vi "Current Loop - NI 9505 (FPGA).vi"() -> ()   [LabVIEW 2012]
doc: "This VI shows an example of how to implement a current loop for use with the NI 9505. The VI consists of a closed loop PI system with PWM generation and error monitoring. The desired load current can be set and the loop will monitor the actual current and adjust the PWM duty cycle until the desired current is reached."
uses:
  <vilib>/LabVIEW Targets/FPGA/cRIO/cRIO-9505/controls.llb/_nicrio_cRIO-9505_DriveStatus.ctl
  <vilib>/Platform/TimedLoop/XDataNode/timing_clust.ctl
  <vilib>/Platform/TimedLoop/XDataNode/nitl_modes.ctl
  <vilib>/Platform/TimedLoop/XDataNode/wakeup.ctl
  <vilib>/LabVIEW Targets/FPGA/cRIO/cRIO-9505/controls.llb/_nicrio_cRIO-9505_DriveDirection.ctl
  <vilib>/rvi/Emulation/niFpgaSctlEmulationRegisterWithScheduler.vi
  <vilib>/rvi/Emulation/niFpgaSctlEmulationScheduler.vi
  <vilib>/rvi/Emulation/niFpgaSctlEmulationGetInTimedLoop.vi
  <vilib>/rvi/eio/common/nirviEmuTemplateMethod_errors.vi
  <vilib>/rvi/Emulation/niFpgaSctlEmulationGlobalWrite.vi
  <vilib>/rvi/eio/common/nirviEmuTemplatePropertyGet_noerrors.vi
  Instance           1 37Saved   Current Loop - NI 9505 (FPGA) .vi
  <vilib>/Platform/TimedLoop/XDataNode/XDataNode.xnode
  <vilib>/eio/EIONode/EIONode.xnode
  <vilib>/eio/EIOMethodNode/EIOMethodNode.xnode
  <vilib>/eio/EIOPropertyNode/EIOPropertyNode.xnode
  <vilib>/Platform/TimedLoop/XDataNode/XDNodeRunTimeDep.lvlib
  <vilib>/rvi/eio/common/nirviEmuTemplatePropertyGet_errors.vi
  <vilib>/rvi/eio/common/nirviEmuTemplatePropertySet_errors.vi
  <vilib>/rvi/eio/common/nirviEmuTemplatePropertySet_noerrors.vi
panel:
  in  "Disable\nDrive":bool
  in  "Enable\nDrive":bool
  out "Temp Fault":bool
  out "Drive Status":T1=enum."Disabled"
  out "Drive Fault":bool
  out "Vsup Present":bool
  in  "Current Loop\nRate (usec)":u32=50
  in  "Current Limit":i16 caption="Setpoint" min=0 max=2047
  in  "Current PI gains":T2={"Proportional Gain"=20, "Integral Gain"=10, "Derivative Gain"=0}
  in  "Current Setpoint":i16 caption="Setpoint"
  in  "Trig AI":bool
  in  "Current Feedback":i16
  out "PWM Duty Cycle":i16
  # "VI Execution\nThis VI should be run using \"Current Loop - NI 9505 (RT).vi\"."
  # "These parameters control the response\nof the current loop. The setpoint is the\ncommanded current and the limit is the\nmaximum current command allowed."
  # "These status controls/indicators are\nused to enable/disable the drive and\nread fault information."
  # "These three controls/indicators are\nused by the individual loops and should\nnot be changed."
  # "Drive Status"
  # "Current Loop Parameters"
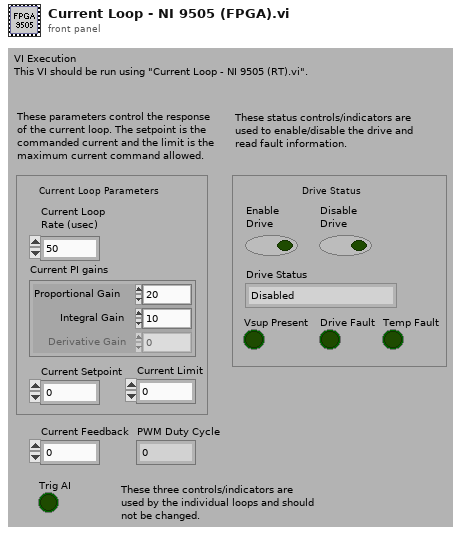
[diagram p1: front panel]
types:
  T1 = typedef "_nicrio_cRIO-9505_DriveStatus.ctl" = enum8{"Enabled", "Disabled", "Disabled by Drive Fault", "Disabled by Temp. Fault", "Disabled by E-Stop", "Unknown"}
  T2 = cluster{"Proportional Gain":i16, "Integral Gain":i16, "Derivative Gain":i16}
  T3 = typedef "XDNodeRunTimeDep.lvlib/timing_clust.ctl" = cluster{"Expected End [f-1]":u64, "Actual End [f-1]":u64, "Finished Late? [f-1]":bool, "Expected End [i-1]":u64, "Actual End [i-1]":u64, "Finished Late? [i-1]":bool, "Expected Start [i]":u64, "Actual Start [i]":u64, "Expected Start [f]":u64, "Actual Start [f]":u64, "Source Name":string, "Structure Name":string, "Period":i64, "Deadline":i64, "Offset":i64, "Start":i64, "Priority":i32, "Timeout":i32, "Mode":T4, "Wakeup Reason":T5, "Error":errorcluster, "Source Type":string, "Secondary Source Type":string, "Global End Time":u64, "Global Start Time":u64, "Frame Duration":u64, "Iteration Duration":u64, "Assigned CPU":i32, "I/O Scan Engine Mode":u32}
  T4 = typedef "XDNodeRunTimeDep.lvlib/nitl_modes.ctl" = enum32{"No Change", "Process missed periods, maintain original phase", "Discard missed periods, maintain original phase", "Process missed periods, ignore original phase", "Discard missed periods, ignore original phase"}
  T5 = typedef "XDNodeRunTimeDep.lvlib/wakeup.ctl" = enum32{"Normal", "Aborted", "Asynchronous wakeup", "Timing source error", "Timed loop error", "Timeout"}
  T6 = typedef "_nicrio_cRIO-9505_DriveDirection.ctl" = enum8{"Clockwise", "Counterclockwise"}
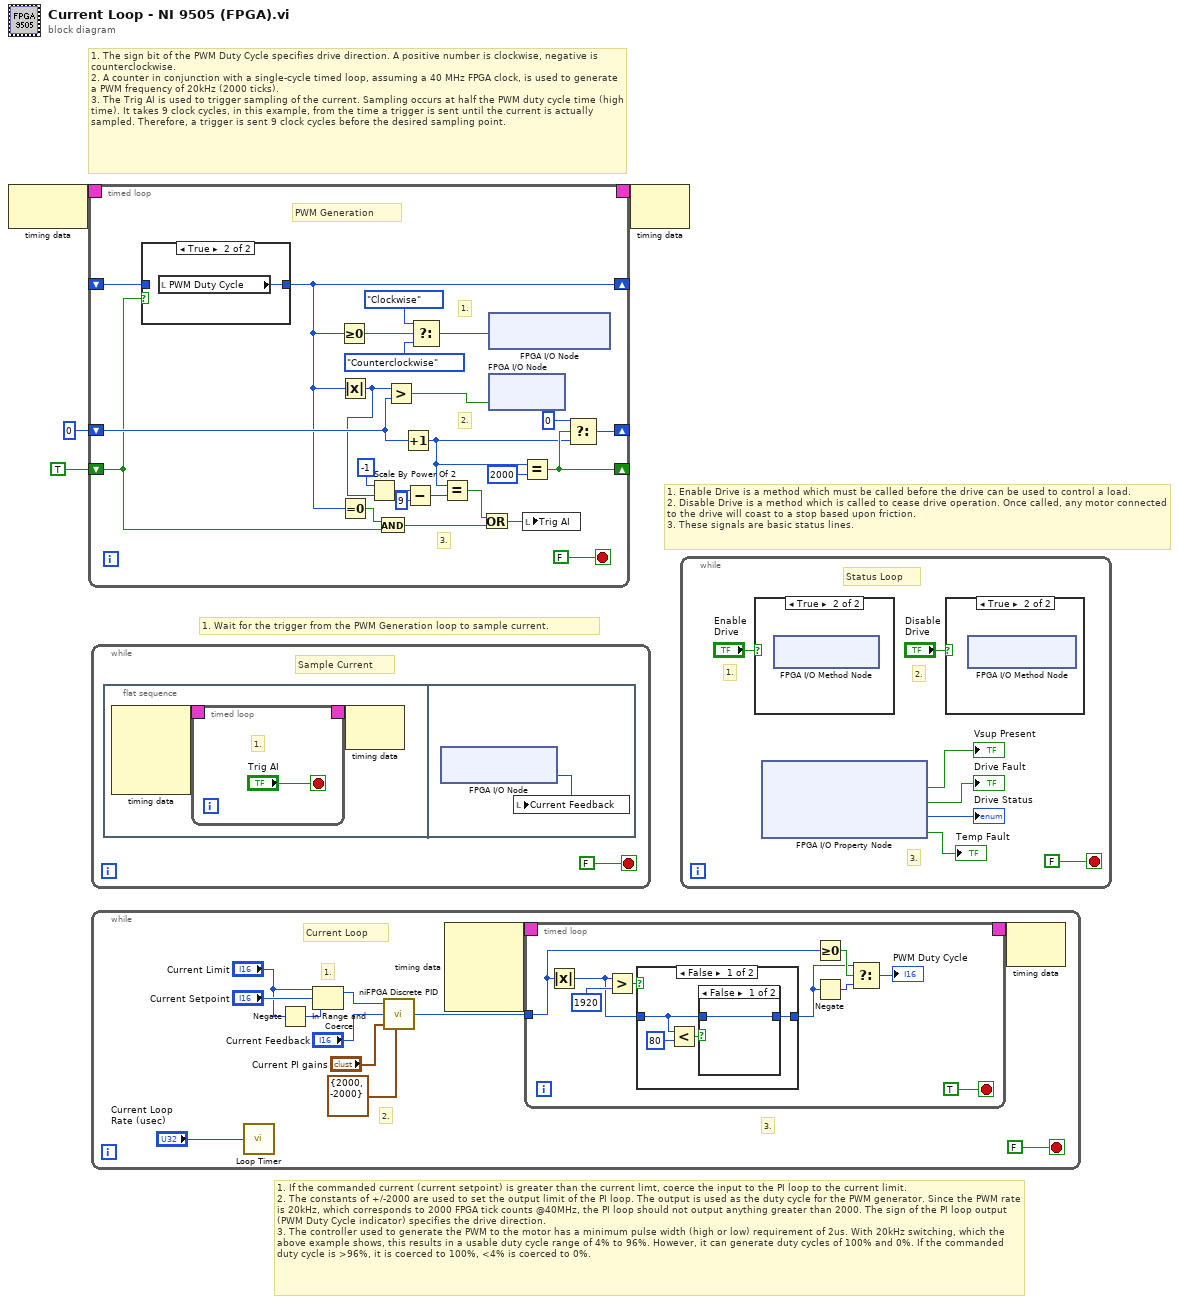
[diagram p0: block diagram]
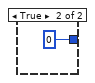
[diagram p5: hidden frame]
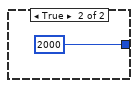
[diagram p6: hidden frame]
diagram:
  # "1. Enable Drive is a method which must be called before the drive can be used to control a load.\n2. Disable Drive is a method which is called to cease drive operation. Once called, any motor connected to the drive will coast to a stop based upon friction.\n3. These signals are basic status lines."
  # "1. Wait for the trigger from the PWM Generation loop to sample current."
  # "1. The sign bit of the PWM Duty Cycle specifies drive direction. A positive number is clockwise, negative is counterclockwise.\n2. A counter in conjunction with a single-cycle timed loop, assuming a 40 MHz FPGA clock, is used to generate a PWM frequency of 20kHz (2000 ticks).\n3. The Trig AI is used to trigger sampling of the current. Sampling occurs at half the PWM duty cycle time (high time). It takes 9 clock cycles, in this example, from the time a trigger is sent until the current is actually sampled. Therefore, a trigger is sent 9 clock cycles before the desired sampling point."
  # "1. If the commanded current (current setpoint) is greater than the current limt, coerce the input to the PI loop to the current limit.\n2. The constants of +/-2000 are used to set the output limit of the PI loop. The output is used as the duty cycle for the PWM generator. Since the PWM rate is 20kHz, which corresponds to 2000 FPGA tick counts @40MHz, the PI loop should not output anything greater than 2000. The sign of the PI loop output (PWM Duty Cycle indicator) specifies the drive direction.\n3. The controller used to generate the PWM to the motor has a minimum pulse width (high or low) requirement of 2us. With 20kHz switching, which the above example shows, this results in a usable duty cycle range of 4% to 96%. However, it can generate duty cycles of 100% and 0%. If the commanded duty cycle is >96%, it is coerced to 100%, <4% is coerced to 0%."
  n1 = node-c288() -> (w4:T3)  [unwired: 1 out]
  n2 = timed-loop {
    timing: w4 -> [_]
    timing-out: [_] -> w3
    shift-right: [w25] -> _
    shift-left: i16 0 -> [w28]
    shift-right: [w24] -> _
    shift-left: TRUE -> [w21]
    shift-right: [w8] -> _
    shift-left: _ -> [w23]
    stop <- FALSE stop-if-true
    # "3."
    # "2."
    # "1."
    # "PWM Generation"
    n3 = case shown="True" w21 {
      tunnel: [w29 w30] -> w8
      tunnel: w23 -> [w29 _]
      frame False {
      }
      frame True {
        n4 = local read "PWM Duty Cycle"() -> (w30:i16)
      }
    }
    n5 = Greater Or Equal To 0?(x=w8) -> (x >= 0?=w17:bool)
    n6 = Absolute Value(x=w8) -> (abs(x)=w6:i16)
    n7 = Equal To 0?(x=w8) -> (x = 0?=w22:bool)
    n8 = Scale By Power Of 2(n=i8 -1, x=w6) -> (x*2^n=w10:i16)
    n9 = And(x=w22, y=w21) -> (x .and. y?=w18:bool)
    n10 = Greater?(x=w6, y=w28) -> (0:w14:bool)
    n11 = Increment(x=w28) -> (x+1=w20:i16)
    n12 = Subtract(x=w10, y=i8 9) -> (x-y=w9:i16)
    n13 = Select(t=_nicrio_cRIO-9505_DriveDirection."Clockwise" ("Drive Direction"), s=w17, f=_nicrio_cRIO-9505_DriveDirection."Counterclockwise" ("Drive Direction")) -> (s? t:f=w13:T6)
    n14 = Equal?(x=w20, y=w9) -> (x = y?=w19:bool)
    n15 = Or(x=w19, y=w18) -> (x .or. y?=w12:bool)
    n16 = xnode "FPGA I/O Node"("Drive Direction"=w13) -> ()  [unwired: 1 in, 1 out]
    n17 = xnode "FPGA I/O Node"("Motor"=w14) -> ()  [unwired: 1 in, 1 out]
    n18 = Equal?(x=w20, y=i16 2000) -> (x = y?=w24:bool)
    n19 = local write "Trig AI"(w12) -> ()
    n20 = Select(t=i16 0, s=w24, f=w20) -> (s? t:f=w25:i16)
  }
  n21 = while {
    stop <- FALSE stop-if-true
    # "Sample Current"
    n22 = flat-sequence {
      frame #0 {
        n23 = node-c288() -> (w35:T3)  [unwired: 4 out]
        n24 = timed-loop {
          timing: w35 -> [_]
          timing-out: [_] -> w34
          stop <- "Trig AI" stop-if-true
          # "1."
        }
        n25 = node-c288(w34) -> ()  [unwired: 1 out]
      }
      frame #1 {
        n26 = xnode "FPGA I/O Node"() -> ("Current Sense"=w41:i16)  [unwired: 1 in, 1 out]
        n27 = local write "Current Feedback"(w41) -> ()
      }
    }
  }
  n28 = while {
    stop <- FALSE stop-if-true
    # "3."
    # "2."
    # "1."
    # "Current Loop"
    n29 = call "Loop Timer"("Count(uSec)"="Current Loop\nRate (usec)") -> ()  [unwired: 1 out]
    n30 = Negate(x="Current Limit") -> (-x=w46:i16)
    n31 = In Range and Coerce(upper limit="Current Limit", x="Current Setpoint", lower limit=w46) -> (coerced(x)=w44:i16)  [unwired: 1 out]
    n32 = call <vilib>:"niFPGA Discrete PID.vi"("setpoint"=w44, "process variable"="Current Feedback", "PID gains (x 2^8)"="Current PI gains", "output range"=cluster{"output high":i16, "output low":i16} {"output high"=2000, "output low"=-2000}) -> ("output"=w50:i16)  [unwired: 1 in, 4 out]
    n33 = node-c288() -> (w49:T3)  [unwired: 4 out]
    n34 = timed-loop {
      timing: w49 -> [_]
      timing-out: [_] -> w48
      tunnel: w50 -> [w56]
      stop <- TRUE stop-if-true
      n35 = Absolute Value(x=w56) -> (abs(x)=w57:i16)
      n36 = Greater?(x=w57, y=i16 1920 ("upper limit")) -> (0:w59:bool)
      n37 = case shown="False" w59 {
        tunnel: [w65 i16 2000 ("upper limit")] -> w58
        tunnel: w57 -> [w63 _]
        frame False {
          n38 = Less?(x=w63, y=i16 80 ("lower limit")) -> (x < y?=w64:bool)
          n39 = case shown="False" w64 {
            tunnel: [w67 i16 0 ("upper limit")] -> w65
            tunnel: w63 -> [w67 _]
            frame False {
            }
            frame True {
            }
          }
        }
        frame True {
        }
      }
      n40 = Greater Or Equal To 0?(x=w56) -> (x >= 0?=w62:bool)
      n41 = Negate(x=w58) -> (-x=w61:i16)
      n42 = Select(t=w58, s=w62, f=w61) -> (s? t:f=→"PWM Duty Cycle":i16)
    }
    n43 = node-c288(w48) -> ()  [unwired: 1 out]
  }
  n44 = node-c288(w3) -> ()  [unwired: 1 out]
  n45 = while {
    stop <- FALSE stop-if-true
    # "3."
    # "2."
    # "1."
    # "Status Loop"
    n46 = case shown="True" "Enable\nDrive" {
      frame False {
      }
      frame True {
        n47 = xnode "FPGA I/O Method Node"() -> ()  [unwired: 1 in, 1 out]
      }
    }
    n48 = xnode "FPGA I/O Property Node"() -> ("Vsup Present"=→"Vsup Present":bool, "Drive Fault"=→"Drive Fault":bool, "Drive Status"=→"Drive Status":T1, "Over Temperature Fault"=→"Temp Fault":bool)  [unwired: 1 in, 1 out]
    n49 = case shown="True" "Disable\nDrive" {
      frame False {
      }
      frame True {
        n50 = xnode "FPGA I/O Method Node"() -> ()  [unwired: 1 in, 1 out]
      }
    }
  }
